vi "Calc Zernike Modes v1.vi"(1 "t":dbl, 2 "r":dbl, 3 "z":i8) -> (0 "zernike":dbl)   [LabVIEW 2018]
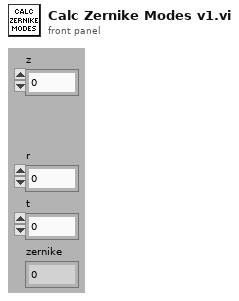
[diagram p1: front panel]
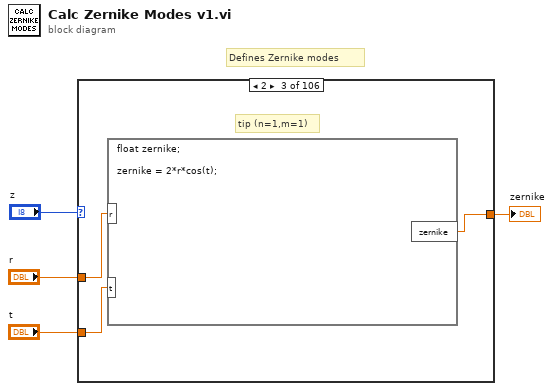
[diagram p0: block diagram]
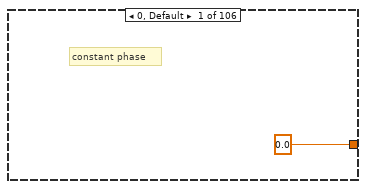
[diagram p2: hidden frame]
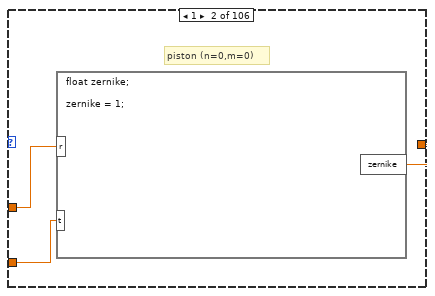
[diagram p3: hidden frame]
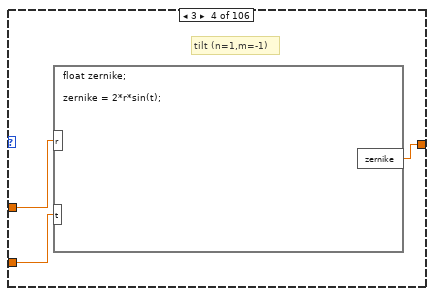
[diagram p4: hidden frame]
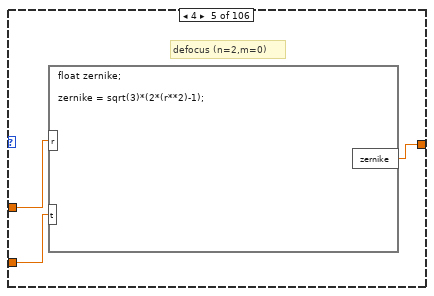
[diagram p5: hidden frame]
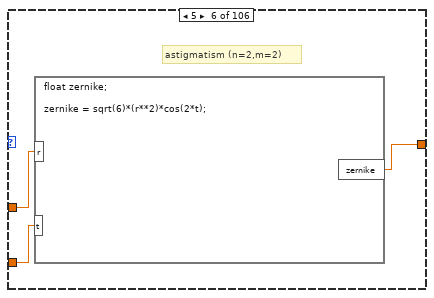
[diagram p6: hidden frame]
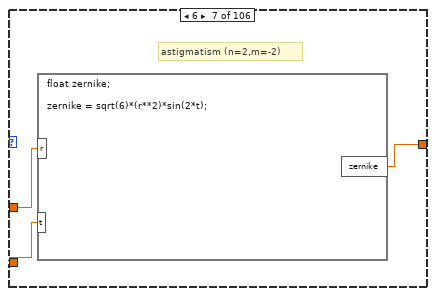
[diagram p7: hidden frame]
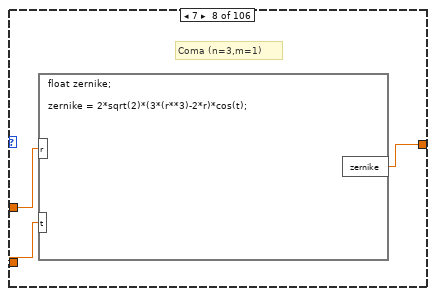
[diagram p8: hidden frame]
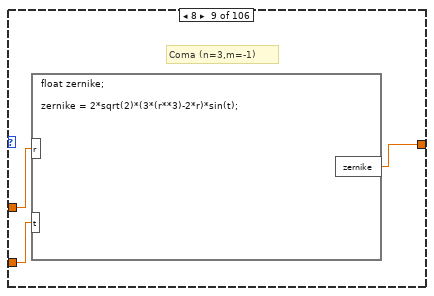
[diagram p9: hidden frame]
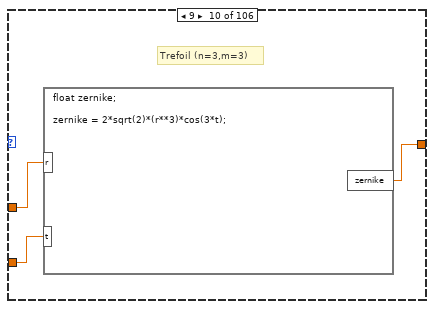
[diagram p10: hidden frame]
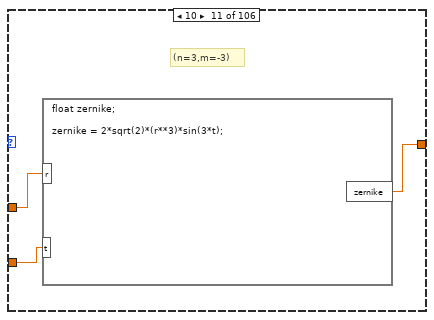
[diagram p11: hidden frame]
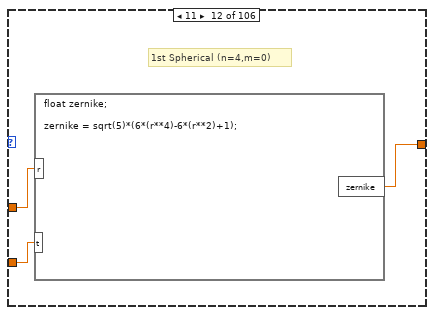
[diagram p12: hidden frame]
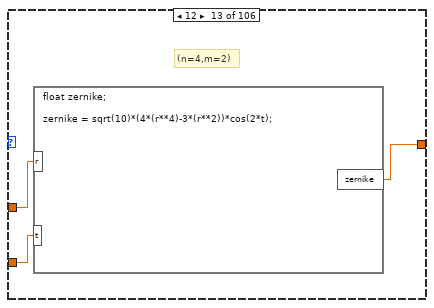
[diagram p13: hidden frame]
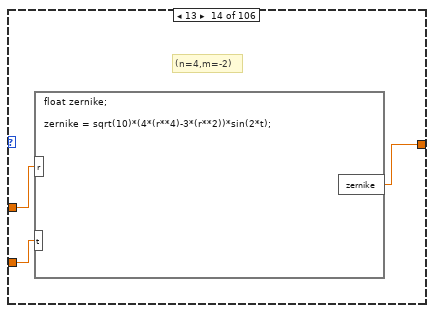
[diagram p14: hidden frame]
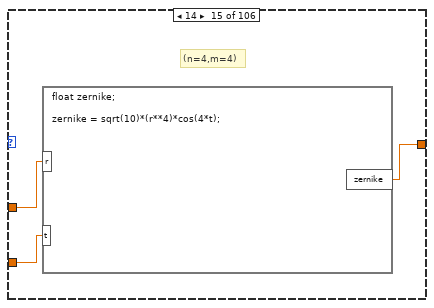
[diagram p15: hidden frame]
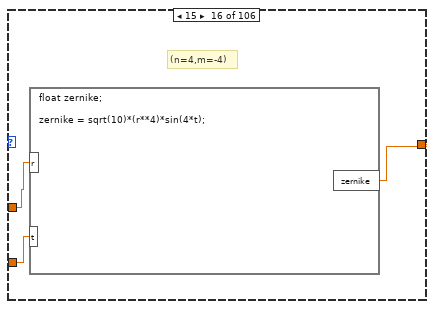
[diagram p16: hidden frame]
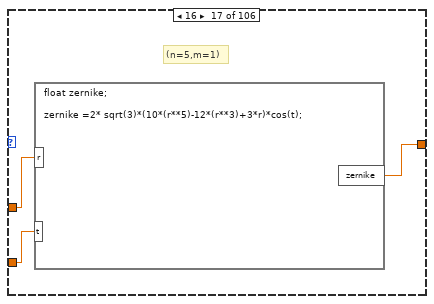
[diagram p17: hidden frame]
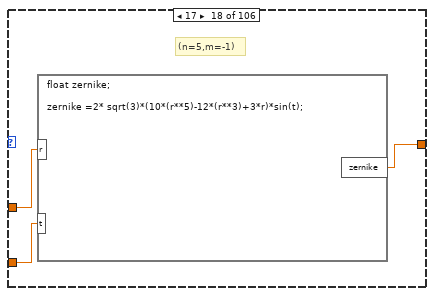
[diagram p18: hidden frame]
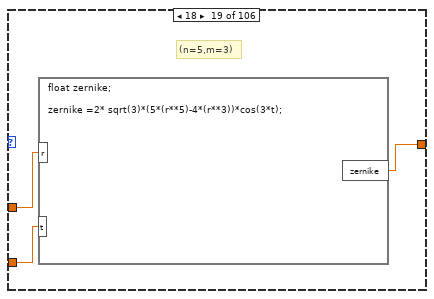
[diagram p19: hidden frame]
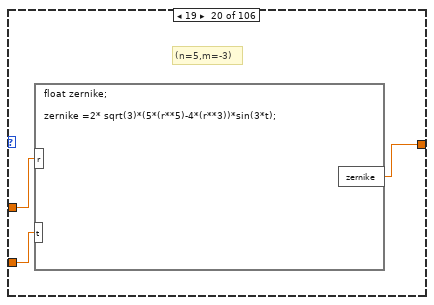
[diagram p20: hidden frame]
diagram:
  # "Defines Zernike modes"
  n1 = case shown="2" "z" {
    tunnel: "r" -> [_ w7 w11 w13 w16 w18 w21 w24 w29 w32 w34 w38 w41 w44 w47 w49 w52 w56 w59 w61 w65 w67 w70 w73 w76 w79 w83 w85 w88 w91 w94 w97 w100 w103 w106 w109 w112 w115 w119 w122 w125 w128 w131 w134 w137 w140 w143 w146 w149 w152 w155 w158 w161 w164 w167 w170 w173 w176 w179 w182 w185 w188 w191 w194 w197 w200 w203 w206 w209 w212 w215 w218 w221 w224 w227 w230 w233 w236 w239 w242 w245 w248 w251 w254 w257 w260 w263 w266 w269 w272 w275 w278 w281 w284 w287 w290 w293 w296 w299 w302 w305 w308 w311 w314 w317 w320]
    tunnel: "t" -> [_ w6 w10 w12 w15 w20 w23 w26 w28 w31 w33 w37 w40 w43 w46 w48 w51 w55 w58 w60 w64 w66 w69 w72 w75 w78 w81 w84 w87 w90 w93 w96 w99 w102 w105 w108 w111 w114 w118 w121 w124 w127 w130 w133 w136 w139 w142 w145 w148 w151 w154 w157 w160 w163 w166 w169 w172 w175 w178 w181 w184 w187 w190 w193 w196 w199 w202 w205 w208 w211 w214 w217 w220 w223 w226 w229 w232 w235 w238 w241 w244 w247 w250 w253 w256 w259 w262 w265 w268 w271 w274 w277 w280 w283 w286 w289 w292 w295 w298 w301 w304 w307 w310 w313 w316 w319]
    tunnel: [0.0 w8 w9 w14 w17 w19 w22 w25 w27 w30 w35 w36 w39 w42 w45 w50 w53 w54 w57 w62 w63 w68 w71 w74 w77 w80 w82 w86 w89 w92 w95 w98 w101 w104 w107 w110 w113 w116 w117 w120 w123 w126 w129 w132 w135 w138 w141 w144 w147 w150 w153 w156 w159 w162 w165 w168 w171 w174 w177 w180 w183 w186 w189 w192 w195 w198 w201 w204 w207 w210 w213 w216 w219 w222 w225 w228 w231 w234 w237 w240 w243 w246 w249 w252 w255 w258 w261 w264 w267 w270 w273 w276 w279 w282 w285 w288 w291 w294 w297 w300 w303 w306 w309 w312 w315 w318] -> w2
    frame 0, Default {
      # "constant phase"
    }
    frame 1 {
      # "piston (n=0,m=0)"
      n2 = formula code="float zernike;\n\nzernike = 1;"("r"=w7, "t"=w6) -> ("zernike"=w8:dbl)
    }
    frame 2 {
      # "tip (n=1,m=1)"
      n3 = formula code="float zernike;\n\nzernike = 2*r*cos(t);"("r"=w11, "t"=w10) -> ("zernike"=w9:dbl)
    }
    frame 3 {
      # "tilt (n=1,m=-1)"
      n4 = formula code="float zernike;\n\nzernike = 2*r*sin(t);"("r"=w13, "t"=w12) -> ("zernike"=w14:dbl)
    }
    frame 4 {
      # "defocus (n=2,m=0)"
      n5 = formula code="float zernike;\n\nzernike = sqrt(3)*(2*(r**2)-1);"("r"=w16, "t"=w15) -> ("zernike"=w17:dbl)
    }
    frame 5 {
      # "astigmatism (n=2,m=2)"
      n6 = formula code="float zernike;\n\nzernike = sqrt(6)*(r**2)*cos(2*t);"("r"=w18, "t"=w20) -> ("zernike"=w19:dbl)
    }
    frame 6 {
      # "astigmatism (n=2,m=-2)"
      n7 = formula code="float zernike;\n\nzernike = sqrt(6)*(r**2)*sin(2*t);"("r"=w21, "t"=w23) -> ("zernike"=w22:dbl)
    }
    frame 7 {
      # "Coma (n=3,m=1)"
      n8 = formula code="float zernike;\n\nzernike = 2*sqrt(2)*(3*(r**3)-2*r)*cos(t);"("r"=w24, "t"=w26) -> ("zernike"=w25:dbl)
    }
    frame 8 {
      # "Coma (n=3,m=-1)"
      n9 = formula code="float zernike;\n\nzernike = 2*sqrt(2)*(3*(r**3)-2*r)*sin(t);"("r"=w29, "t"=w28) -> ("zernike"=w27:dbl)
    }
    frame 9 {
      # "Trefoil (n=3,m=3)"
      n10 = formula code="float zernike;\n\nzernike = 2*sqrt(2)*(r**3)*cos(3*t);"("r"=w32, "t"=w31) -> ("zernike"=w30:dbl)
    }
    frame 10 {
      # "(n=3,m=-3)"
      n11 = formula code="float zernike;\n\nzernike = 2*sqrt(2)*(r**3)*sin(3*t);"("r"=w34, "t"=w33) -> ("zernike"=w35:dbl)
    }
    frame 11 {
      # "1st Spherical (n=4,m=0)"
      n12 = formula code="float zernike;\n\nzernike = sqrt(5)*(6*(r**4)-6*(r**2)+1);"("r"=w38, "t"=w37) -> ("zernike"=w36:dbl)
    }
    frame 12 {
      # "(n=4,m=2)"
      n13 = formula code="float zernike;\n\nzernike = sqrt(10)*(4*(r**4)-3*(r**2))*cos(2*t);"("r"=w41, "t"=w40) -> ("zernike"=w39:dbl)
    }
    frame 13 {
      # "(n=4,m=-2)"
      n14 = formula code="float zernike;\n\nzernike = sqrt(10)*(4*(r**4)-3*(r**2))*sin(2*t);"("r"=w44, "t"=w43) -> ("zernike"=w42:dbl)
    }
    frame 14 {
      # "(n=4,m=4)"
      n15 = formula code="float zernike;\n\nzernike = sqrt(10)*(r**4)*cos(4*t);"("r"=w47, "t"=w46) -> ("zernike"=w45:dbl)
    }
    frame 15 {
      # "(n=4,m=-4)"
      n16 = formula code="float zernike;\n\nzernike = sqrt(10)*(r**4)*sin(4*t);"("r"=w49, "t"=w48) -> ("zernike"=w50:dbl)
    }
    frame 16 {
      # "(n=5,m=1)"
      n17 = formula code="float zernike;\n\nzernike =2* sqrt(3)*(10*(r**5)-12*(r**3)+3*r)*cos(t);"("r"=w52, "t"=w51) -> ("zernike"=w53:dbl)
    }
    frame 17 {
      # "(n=5,m=-1)"
      n18 = formula code="float zernike;\n\nzernike =2* sqrt(3)*(10*(r**5)-12*(r**3)+3*r)*sin(t);"("r"=w56, "t"=w55) -> ("zernike"=w54:dbl)
    }
    frame 18 {
      # "(n=5,m=3)"
      n19 = formula code="float zernike;\n\nzernike =2* sqrt(3)*(5*(r**5)-4*(r**3))*cos(3*t);"("r"=w59, "t"=w58) -> ("zernike"=w57:dbl)
    }
    frame 19 {
      # "(n=5,m=-3)"
      n20 = formula code="float zernike;\n\nzernike =2* sqrt(3)*(5*(r**5)-4*(r**3))*sin(3*t);"("r"=w61, "t"=w60) -> ("zernike"=w62:dbl)
    }
    frame 20 {
      # "(n=5,m=5)"
      n21 = formula code="float zernike;\n\nzernike =2* sqrt(3)*(r**5)*cos(5*t);"("r"=w65, "t"=w64) -> ("zernike"=w63:dbl)
    }
    frame 21 {
      # "(n=5,m=5)"
      n22 = formula code="float zernike;\n\nzernike =2* sqrt(3)*(r**5)*sin(5*t);"("r"=w67, "t"=w66) -> ("zernike"=w68:dbl)
    }
    frame 22 {
      # "(n=6,m=0)"
      n23 = formula code="float zernike;\n\nzernike = sqrt(7)*(20*(r**6)-30*(r**4)+12*(r**2)-1);"("r"=w70, "t"=w69) -> ("zernike"=w71:dbl)
    }
    frame 23 {
      # "(n=6,m=2)"
      n24 = formula code="float zernike;\n\nzernike = sqrt(14)*(15*(r**6)-20*(r**4)+6*(r**2))*cos(2*t);"("r"=w73, "t"=w72) -> ("zernike"=w74:dbl)
    }
    frame 24 {
      # "(n=6,m=-2)"
      n25 = formula code="float zernike;\n\nzernike = sqrt(14)*(15*(r**6)-20*(r**4)+6*(r**2))*sin(2*t);"("r"=w76, "t"=w75) -> ("zernike"=w77:dbl)
    }
    frame 25 {
      # "(n=6,m=4)"
      n26 = formula code="float zernike;\n\nzernike = sqrt(14)*(6*(r**6)-5*(r**4))*cos(4*t);"("r"=w79, "t"=w78) -> ("zernike"=w80:dbl)
    }
    frame 26 {
      # "(n=6,m=-4)"
      n27 = formula code="float zernike;\n\nzernike = sqrt(14)*(6*(r**6)-5*(r**4))*sin(4*t);"("r"=w83, "t"=w81) -> ("zernike"=w82:dbl)
    }
    frame 27 {
      # "(n=6,m=6)"
      n28 = formula code="float zernike;\n\nzernike = sqrt(14)*((r**6))*cos(6*t);"("r"=w85, "t"=w84) -> ("zernike"=w86:dbl)
    }
    frame 28 {
      # "(n=6,m=-6)"
      n29 = formula code="float zernike;\n\nzernike = sqrt(14)*((r**6))*sin(6*t);"("r"=w88, "t"=w87) -> ("zernike"=w89:dbl)
    }
    frame 29 {
      # "(n=7,m=1)"
      n30 = formula code="float zernike;\n\nzernike = 4*(35*(r**7)-60*(r**5)+30*(r**3)-4*r)*cos(t);"("r"=w91, "t"=w90) -> ("zernike"=w92:dbl)
    }
    frame 30 {
      # "(n=7,m=-1)"
      n31 = formula code="float zernike;\n\nzernike = 4*(35*(r**7)-60*(r**5)+30*(r**3)-4*r)*sin(t);"("r"=w94, "t"=w93) -> ("zernike"=w95:dbl)
    }
    frame 31 {
      # "(n=7,m=3)"
      n32 = formula code="float zernike;\n\nzernike = 4*(21*(r**7)-30*(r**5)+10*(r**3))*cos(3*t);"("r"=w97, "t"=w96) -> ("zernike"=w98:dbl)
    }
    frame 32 {
      # "(n=7,m=-3)"
      n33 = formula code="float zernike;\n\nzernike = 4*(21*(r**7)-30*(r**5)+10*(r**3))*sin(3*t);"("r"=w100, "t"=w99) -> ("zernike"=w101:dbl)
    }
    frame 33 {
      # "(n=7,m=5)"
      n34 = formula code="float zernike;\n\nzernike = 4*(7*(r**7)-6*(r**5))*cos(5*t);"("r"=w103, "t"=w102) -> ("zernike"=w104:dbl)
    }
    frame 34 {
      # "(n=7,m=-5)"
      n35 = formula code="float zernike;\n\nzernike = 4*(7*(r**7)-6*(r**5))*sin(5*t);"("r"=w106, "t"=w105) -> ("zernike"=w107:dbl)
    }
    frame 35 {
      # "(n=7,m=7)"
      n36 = formula code="float zernike;\n\nzernike = 4*((r**7))*cos(7*t);"("r"=w109, "t"=w108) -> ("zernike"=w110:dbl)
    }
    frame 36 {
      # "(n=7,m=-7)"
      n37 = formula code="float zernike;\n\nzernike = 4*((r**7))*sin(7*t);"("r"=w112, "t"=w111) -> ("zernike"=w113:dbl)
    }
    frame 37 {
      # "(n=8,m=0)"
      n38 = formula code="float zernike;\n\nzernike = 3*(70*(r**8)-140*(r**6)+90*(r**4)-20*(r**2)+1);"("r"=w115, "t"=w114) -> ("zernike"=w116:dbl)
    }
    frame 38 {
      # "(n=8,m=2)"
      n39 = formula code="float zernike;\n\nzernike = 3*sqrt(2)*(56*(r**8)-105*(r**6)+60*(r**4)-10*(r**2))*cos(2*t);"("r"=w119, "t"=w118) -> ("zernike"=w117:dbl)
    }
    frame 39 {
      # "(n=8,m=-2)"
      n40 = formula code="float zernike;\n\nzernike = 3*sqrt(2)*(56*(r**8)-105*(r**6)+60*(r**4)-10*(r**2))*sin(2*t);"("r"=w122, "t"=w121) -> ("zernike"=w120:dbl)
    }
    frame 40 {
      # "(n=8,m=4)"
      n41 = formula code="float zernike;\n\nzernike = 3*sqrt(2)*(28*(r**8)-42*(r**6)+15*(r**4))*cos(4*t);"("r"=w125, "t"=w124) -> ("zernike"=w123:dbl)
    }
    frame 41 {
      # "(n=8,m=-4)"
      n42 = formula code="float zernike;\n\nzernike = 3*sqrt(2)*(28*(r**8)-42*(r**6)+15*(r**4))*sin(4*t);"("r"=w128, "t"=w127) -> ("zernike"=w126:dbl)
    }
    frame 42 {
      # "(n=8,m=6)"
      n43 = formula code="float zernike;\n\nzernike = 3*sqrt(2)*(8*(r**8)-7*(r**6))*cos(6*t);"("r"=w131, "t"=w130) -> ("zernike"=w129:dbl)
    }
    frame 43 {
      # "(n=8,m=-6)"
      n44 = formula code="float zernike;\n\nzernike = 3*sqrt(2)*(8*(r**8)-7*(r**6))*sin(6*t);"("r"=w134, "t"=w133) -> ("zernike"=w132:dbl)
    }
    frame 44 {
      # "(n=8,m=8)"
      n45 = formula code="float zernike;\n\nzernike = 3*sqrt(2)*((r**8))*cos(8*t);"("r"=w137, "t"=w136) -> ("zernike"=w135:dbl)
    }
    frame 45 {
      # "(n=8,m=-8)"
      n46 = formula code="float zernike;\n\nzernike = 3*sqrt(2)*((r**8))*sin(8*t);"("r"=w140, "t"=w139) -> ("zernike"=w138:dbl)
    }
    frame 46 {
      # "(n=9,m=1)"
      n47 = formula code="float zernike;\n\nzernike = 2*sqrt(5)*(126*(r**9)-280*(r**7)+210*(r**5)-60*(r**3)+5*r)*cos(t);"("r"=w143, "t"=w142) -> ("zernike"=w141:dbl)
    }
    frame 47 {
      # "(n=9,m=-1)"
      n48 = formula code="float zernike;\n\nzernike = 2*sqrt(5)*(126*(r**9)-280*(r**7)+210*(r**5)-60*(r**3)+5*r)*sin(t);"("r"=w146, "t"=w145) -> ("zernike"=w144:dbl)
    }
    frame 48 {
      # "(n=9,m=3)"
      n49 = formula code="float zernike;\n\nzernike = 2*sqrt(5)*(84*(r**9)-168*(r**7)+105*(r**5)-20*(r**3))*cos(3*t);"("r"=w149, "t"=w148) -> ("zernike"=w147:dbl)
    }
    frame 49 {
      # "(n=9,m=-3)"
      n50 = formula code="float zernike;\n\nzernike = 2*sqrt(5)*(84*(r**9)-168*(r**7)+105*(r**5)-20*(r**3))*sin(3*t);"("r"=w152, "t"=w151) -> ("zernike"=w150:dbl)
    }
    frame 50 {
      # "(n=9,m=5)"
      n51 = formula code="float zernike;\n\nzernike = 2*sqrt(5)*(36*(r**9)-56*(r**7)+21*(r**5))*cos(5*t);"("r"=w155, "t"=w154) -> ("zernike"=w153:dbl)
    }
    frame 51 {
      # "(n=9,m=-5)"
      n52 = formula code="float zernike;\n\nzernike = 2*sqrt(5)*(36*(r**9)-56*(r**7)+21*(r**5))*sin(5*t);"("r"=w158, "t"=w157) -> ("zernike"=w156:dbl)
    }
    frame 52 {
      # "(n=9,m=7)"
      n53 = formula code="float zernike;\n\nzernike = 2*sqrt(5)*(9*(r**9)-8*(r**7))*cos(7*t);"("r"=w161, "t"=w160) -> ("zernike"=w159:dbl)
    }
    frame 53 {
      # "(n=9,m=-7)"
      n54 = formula code="float zernike;\n\nzernike = 2*sqrt(5)*(9*(r**9)-8*(r**7))*sin(7*t);"("r"=w164, "t"=w163) -> ("zernike"=w162:dbl)
    }
    frame 54 {
      # "(n=9,m=9)"
      n55 = formula code="float zernike;\n\nzernike = 2*sqrt(5)*((r**9))*cos(9*t);"("r"=w167, "t"=w166) -> ("zernike"=w165:dbl)
    }
    frame 55 {
      # "(n=9,m=-9)"
      n56 = formula code="float zernike;\n\nzernike = 2*sqrt(5)*((r**9))*sin(9*t);"("r"=w170, "t"=w169) -> ("zernike"=w168:dbl)
    }
    frame 56 {
      # "(n=10,m=0)"
      n57 = formula code="float zernike;\n\nzernike = sqrt(11)*(252*(r**10)-630*(r**8)+560*(r**6)-210*(r**4)+30*(r**2)-1);"("r"=w173, "t"=w172) -> ("zernike"=w171:dbl)
    }
    frame 57 {
      # "(n=10,m=2)"
      n58 = formula code="float zernike;\n\nzernike = sqrt(22)*(210*(r**10)-504*(r**8)+420*(r**6)-140*(r**4)+15*(r**2))*cos(2*t);"("r"=w176, "t"=w175) -> ("zernike"=w174:dbl)
    }
    frame 58 {
      # "(n=10,m=-2)"
      n59 = formula code="float zernike;\n\nzernike = sqrt(22)*(210*(r**10)-504*(r**8)+420*(r**6)-140*(r**4)+15*(r**2))*sin(2*t);"("r"=w179, "t"=w178) -> ("zernike"=w177:dbl)
    }
    frame 59 {
      # "(n=10,m=4)"
      n60 = formula code="float zernike;\n\nzernike = sqrt(22)*(120*(r**10)-252*(r**8)+168*(r**6)-35*(r**4))*cos(4*t);"("r"=w182, "t"=w181) -> ("zernike"=w180:dbl)
    }
    frame 60 {
      # "(n=10,m=-4)"
      n61 = formula code="float zernike;\n\nzernike = sqrt(22)*(120*(r**10)-252*(r**8)+168*(r**6)-35*(r**4))*sin(4*t);"("r"=w185, "t"=w184) -> ("zernike"=w183:dbl)
    }
    frame 61 {
      # "(n=10,m=6)"
      n62 = formula code="float zernike;\n\nzernike = sqrt(22)*(45*(r**10)-72*(r**8)+28*(r**6))*cos(6*t);"("r"=w188, "t"=w187) -> ("zernike"=w186:dbl)
    }
    frame 62 {
      # "(n=10,m=-6)"
      n63 = formula code="float zernike;\n\nzernike = sqrt(22)*(45*(r**10)-72*(r**8)+28*(r**6))*sin(6*t);"("r"=w191, "t"=w190) -> ("zernike"=w189:dbl)
    }
    frame 63 {
      # "(n=10,m=8)"
      n64 = formula code="float zernike;\n\nzernike = sqrt(22)*(10*(r**10)-9*(r**8))*cos(8*t);"("r"=w194, "t"=w193) -> ("zernike"=w192:dbl)
    }
    frame 64 {
      # "(n=10,m=-8)"
      n65 = formula code="float zernike;\n\nzernike = sqrt(22)*(10*(r**10)-9*(r**8))*sin(8*t);"("r"=w197, "t"=w196) -> ("zernike"=w195:dbl)
    }
    frame 65 {
      # "(n=10,m=10)"
      n66 = formula code="float zernike;\n\nzernike = sqrt(22)*((r**10))*cos(10*t);"("r"=w200, "t"=w199) -> ("zernike"=w198:dbl)
    }
    frame 66 {
      # "(n=10,m=10)"
      n67 = formula code="float zernike;\n\nzernike = sqrt(22)*((r**10))*sin(10*t);"("r"=w203, "t"=w202) -> ("zernike"=w201:dbl)
    }
    frame 67 {
      # "(n=11,m=1)"
      n68 = formula code="float zernike;\n\nzernike = 2*sqrt(6)*(462*(r**11)-1260*(r**9)+1260*(r**7)-560*(r**5)+105*(r**3)-6*r)*cos(t);"("r"=w206, "t"=w205) -> ("zernike"=w204:dbl)
    }
    frame 68 {
      # "(n=11,m=-1)"
      n69 = formula code="float zernike;\n\nzernike = 2*sqrt(6)*(462*(r**11)-1260*(r**9)+1260*(r**7)-560*(r**5)+105*(r**3)-6*r)*sin(t);"("r"=w209, "t"=w208) -> ("zernike"=w207:dbl)
    }
    frame 69 {
      # "(n=11,m=3)"
      n70 = formula code="float zernike;\n\nzernike = 2*sqrt(6)*(330*(r**11)-840*(r**9)+756*(r**7)-280*(r**5)+35*(r**3))*cos(3*t);"("r"=w212, "t"=w211) -> ("zernike"=w210:dbl)
    }
    frame 70 {
      # "(n=11,m=-3)"
      n71 = formula code="float zernike;\n\nzernike = 2*sqrt(6)*(330*(r**11)-840*(r**9)+756*(r**7)-280*(r**5)+35*(r**3))*sin(3*t);"("r"=w215, "t"=w214) -> ("zernike"=w213:dbl)
    }
    frame 71 {
      # "(n=11,m=5)"
      n72 = formula code="float zernike;\n\nzernike = 2*sqrt(6)*(165*(r**11)-360*(r**9)+252*(r**7)-56*(r**5))*cos(5*t);"("r"=w218, "t"=w217) -> ("zernike"=w216:dbl)
    }
    frame 72 {
      # "(n=11,m=-5)"
      n73 = formula code="float zernike;\n\nzernike = 2*sqrt(6)*(165*(r**11)-360*(r**9)+252*(r**7)-56*(r**5))*sin(5*t);"("r"=w221, "t"=w220) -> ("zernike"=w219:dbl)
    }
    frame 73 {
      # "(n=11,m=7)"
      n74 = formula code="float zernike;\n\nzernike = 2*sqrt(6)*(55*(r**11)-90*(r**9)+36*(r**7))*cos(7*t);"("r"=w224, "t"=w223) -> ("zernike"=w222:dbl)
    }
    frame 74 {
      # "(n=11,m=-7)"
      n75 = formula code="float zernike;\n\nzernike = 2*sqrt(6)*(55*(r**11)-90*(r**9)+36*(r**7))*sin(7*t);"("r"=w227, "t"=w226) -> ("zernike"=w225:dbl)
    }
    frame 75 {
      # "(n=11,m=9)"
      n76 = formula code="float zernike;\n\nzernike = 2*sqrt(6)*(11*(r**11)-10*(r**9))*cos(9*t);"("r"=w230, "t"=w229) -> ("zernike"=w228:dbl)
    }
    frame 76 {
      # "(n=11,m=-9)"
      n77 = formula code="float zernike;\n\nzernike = 2*sqrt(6)*(11*(r**11)-10*(r**9))*sin(9*t);"("r"=w233, "t"=w232) -> ("zernike"=w231:dbl)
    }
    frame 77 {
      # "(n=11,m=11)"
      n78 = formula code="float zernike;\n\nzernike = 2*sqrt(6)*((r**11))*cos(11*t);"("r"=w236, "t"=w235) -> ("zernike"=w234:dbl)
    }
    frame 78 {
      # "(n=11,m=-11)"
      n79 = formula code="float zernike;\n\nzernike = 2*sqrt(6)*((r**11))*sin(11*t);"("r"=w239, "t"=w238) -> ("zernike"=w237:dbl)
    }
    frame 79 {
      # "(n=12,m=0)"
      n80 = formula code="float zernike;\n\nzernike = sqrt(13)*(924*(r**12)-2772*(r**10)+3150*(r**8)-1680*(r**6)+420*(r**4)-42*(r**2)+1);"("r"=w242, "t"=w241) -> ("zernike"=w240:dbl)
    }
    frame 80 {
      # "(n=12,m=2)"
      n81 = formula code="float zernike;\n\nzernike = sqrt(26)*(792*(r**12)-2310*(r**10)+2520*(r**8)-1260*(r**6)+280*(r**4)-21*(r**2))*cos(2*t);"("r"=w245, "t"=w244) -> ("zernike"=w243:dbl)
    }
    frame 81 {
      # "(n=12,m=-2)"
      n82 = formula code="float zernike;\n\nzernike = sqrt(26)*(792*(r**12)-2310*(r**10)+2520*(r**8)-1260*(r**6)+280*(r**4)-21*(r**2))*sin(2*t);"("r"=w248, "t"=w247) -> ("zernike"=w246:dbl)
    }
    frame 82 {
      # "(n=12,m=4)"
      n83 = formula code="float zernike;\n\nzernike = sqrt(26)*(495*(r**12)-1320*(r**10)+1260*(r**8)-504*(r**6)+70*(r**4))*cos(4*t);"("r"=w251, "t"=w250) -> ("zernike"=w249:dbl)
    }
    frame 83 {
      # "(n=12,m=-4)"
      n84 = formula code="float zernike;\n\nzernike = sqrt(26)*(495*(r**12)-1320*(r**10)+1260*(r**8)-504*(r**6)+70*(r**4))*sin(4*t);"("r"=w254, "t"=w253) -> ("zernike"=w252:dbl)
    }
    frame 84 {
      # "(n=12,m=6)"
      n85 = formula code="float zernike;\n\nzernike = sqrt(26)*(220*(r**12)-495*(r**10)+360*(r**8)-84*(r**6))*cos(6*t);"("r"=w257, "t"=w256) -> ("zernike"=w255:dbl)
    }
    frame 85 {
      # "(n=12,m=-6)"
      n86 = formula code="float zernike;\n\nzernike = sqrt(26)*(220*(r**12)-495*(r**10)+360*(r**8)-84*(r**6))*sin(6*t);"("r"=w260, "t"=w259) -> ("zernike"=w258:dbl)
    }
    frame 86 {
      # "(n=12,m=8)"
      n87 = formula code="float zernike;\n\nzernike = sqrt(26)*(66*(r**12)-110*(r**10)+45*(r**8))*cos(8*t);"("r"=w263, "t"=w262) -> ("zernike"=w261:dbl)
    }
    frame 87 {
      # "(n=12,m=-8)"
      n88 = formula code="float zernike;\n\nzernike = sqrt(26)*(66*(r**12)-110*(r**10)+45*(r**8))*sin(8*t);"("r"=w266, "t"=w265) -> ("zernike"=w264:dbl)
    }
    frame 88 {
      # "(n=12,m=10)"
      n89 = formula code="float zernike;\n\nzernike = sqrt(26)*(12*(r**12)-11*(r**10))*cos(10*t);"("r"=w269, "t"=w268) -> ("zernike"=w267:dbl)
    }
    frame 89 {
      # "(n=12,m=10)"
      n90 = formula code="float zernike;\n\nzernike = sqrt(26)*(12*(r**12)-11*(r**10))*sin(10*t);"("r"=w272, "t"=w271) -> ("zernike"=w270:dbl)
    }
    frame 90 {
      # "(n=12,m=12)"
      n91 = formula code="float zernike;\n\nzernike = sqrt(26)*((r**12))*cos(12*t);"("r"=w275, "t"=w274) -> ("zernike"=w273:dbl)
    }
    frame 91 {
      # "(n=12,m=-12)"
      n92 = formula code="float zernike;\n\nzernike = sqrt(26)*((r**12))*sin(12*t);"("r"=w278, "t"=w277) -> ("zernike"=w276:dbl)
    }
    frame 92 {
      # "(n=13,m=1)"
      n93 = formula code="float zernike;\n\nzernike = 2*sqrt(7)*(1716*(r**13)-5544*(r**11)+6930*(r**9)-4200*(r**7)+1260*(r**5)-168*(r**3)+7*r)*cos(t);"("r"=w281, "t"=w280) -> ("zernike"=w279:dbl)
    }
    frame 93 {
      # "(n=13,m=-1)"
      n94 = formula code="float zernike;\n\nzernike = 2*sqrt(7)*(1716*(r**13)-5544*(r**11)+6930*(r**9)-4200*(r**7)+1260*(r**5)-168*(r**3)+7*r)*sin(t);"("r"=w284, "t"=w283) -> ("zernike"=w282:dbl)
    }
    frame 94 {
      # "(n=13,m=3)"
      n95 = formula code="float zernike;\n\nzernike = 2*sqrt(7)*(1287*(r**13)-3960*(r**11)+4620*(r**9)-2520*(r**7)+630*(r**5)-56*(r**3))*cos(3*t);"("r"=w287, "t"=w286) -> ("zernike"=w285:dbl)
    }
    frame 95 {
      # "(n=13,m=-3)"
      n96 = formula code="float zernike;\n\nzernike = 2*sqrt(7)*(1287*(r**13)-3960*(r**11)+4620*(r**9)-2520*(r**7)+630*(r**5)-56*(r**3))*sin(3*t);"("r"=w290, "t"=w289) -> ("zernike"=w288:dbl)
    }
    frame 96 {
      # "(n=13,m=5)"
      n97 = formula code="float zernike;\n\nzernike = 2*sqrt(7)*(715*(r**13)-1980*(r**11)+1980*(r**9)-840*(r**7)+126*(r**5))*cos(5*t);"("r"=w293, "t"=w292) -> ("zernike"=w291:dbl)
    }
    frame 97 {
      # "(n=13,m=-5)"
      n98 = formula code="float zernike;\n\nzernike = 2*sqrt(7)*(715*(r**13)-1980*(r**11)+1980*(r**9)-840*(r**7)+126*(r**5))*sin(5*t);"("r"=w296, "t"=w295) -> ("zernike"=w294:dbl)
    }
    frame 98 {
      # "(n=13,m=7)"
      n99 = formula code="float zernike;\n\nzernike = 2*sqrt(7)*(286*(r**13)-660*(r**11)+495*(r**9)-120*(r**7))*cos(7*t);"("r"=w299, "t"=w298) -> ("zernike"=w297:dbl)
    }
    frame 99 {
      # "(n=13,m=-7)"
      n100 = formula code="float zernike;\n\nzernike = 2*sqrt(7)*(286*(r**13)-660*(r**11)+495*(r**9)-120*(r**7))*sin(7*t);"("r"=w302, "t"=w301) -> ("zernike"=w300:dbl)
    }
    frame 100 {
      # "(n=13,m=9)"
      n101 = formula code="float zernike;\n\nzernike = 2*sqrt(7)*(78*(r**13)-132*(r**11)+55*(r**9))*cos(9*t);"("r"=w305, "t"=w304) -> ("zernike"=w303:dbl)
    }
    frame 101 {
      # "(n=13,m=-9)"
      n102 = formula code="float zernike;\n\nzernike = 2*sqrt(7)*(78*(r**13)-132*(r**11)+55*(r**9))*sin(9*t);"("r"=w308, "t"=w307) -> ("zernike"=w306:dbl)
    }
    frame 102 {
      # "(n=13,m=11)"
      n103 = formula code="float zernike;\n\nzernike = 2*sqrt(7)*(13*(r**13)-12*(r**11))*cos(11*t);"("r"=w311, "t"=w310) -> ("zernike"=w309:dbl)
    }
    frame 103 {
      # "(n=13,m=-11)"
      n104 = formula code="float zernike;\n\nzernike = 2*sqrt(7)*(13*(r**13)-12*(r**11))*sin(11*t);"("r"=w314, "t"=w313) -> ("zernike"=w312:dbl)
    }
    frame 104 {
      # "(n=13,m=-13)"
      n105 = formula code="float zernike;\n\nzernike = 2*sqrt(7)*((r**13))*cos(13*t);"("r"=w317, "t"=w316) -> ("zernike"=w315:dbl)
    }
    frame 105 {
      # "(n=13,m=13)"
      n106 = formula code="float zernike;\n\nzernike = 2*sqrt(7)*((r**13))*sin(13*t);"("r"=w320, "t"=w319) -> ("zernike"=w318:dbl)
    }
  }
  "zernike" <- w2
